vi "Result.Measurement, Screen for Fail or Error.vi"(10 "Meas":T1[](array[typedef]) {"Status" items=["LOG", "PASS", "FAIL", "ERROR"]}, 11 "ResultState In":T3={"State"=enum."Failing", "Code"=0, "Description"=""}) -> (3 "ResultState Out":T3={"State"=enum."Failing", "Code"=0, "Description"=""})   [LabVIEW 2024]
uses:
  <vilib>/KATE/SeqMgr/SeqMgr.Result Info.ctl
  <vilib>/KATE/SeqMgr/SeqMgr.Result State Enum.ctl
  Result.Measurement Item.ctl
  Result.Measurement and Attribute Item Status.ctl
  <vilib>/KATE/SeqMgr/SeqMgr.lvlib
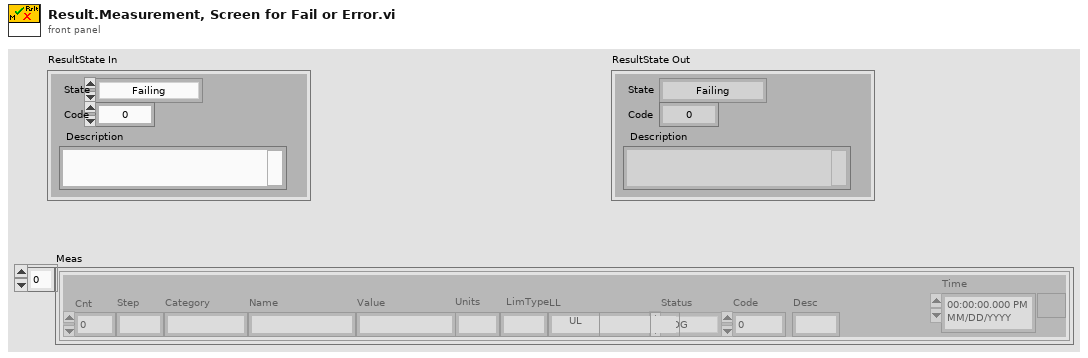
[diagram p1: front panel]
types:
  T1 = typedef "Result.Measurement Item.ctl" = cluster{"Cnt":i32, "Step":string, "Category":string, "Name":string, "Value":string, "Units":string, "LimType":string, "LL":string, "UL":string, "Status":T2, "Code":i32, "Desc":string, "Time":timestamp}
  T2 = typedef "Result.Measurement and Attribute Item Status.ctl" = i32
  T3 = typedef "KATE_Lib.lvlib/SeqMgr.lvlib/SeqMgr.Result Info.ctl" = cluster{"State":T4, "Code":i32, "Description":string}
  T4 = typedef "KATE_Lib.lvlib/SeqMgr.lvlib/SeqMgr.Result State Enum.ctl" = enum16{"None", "Passing", "Failing", "PASS", "FAIL", "ABORT", "ERROR"}
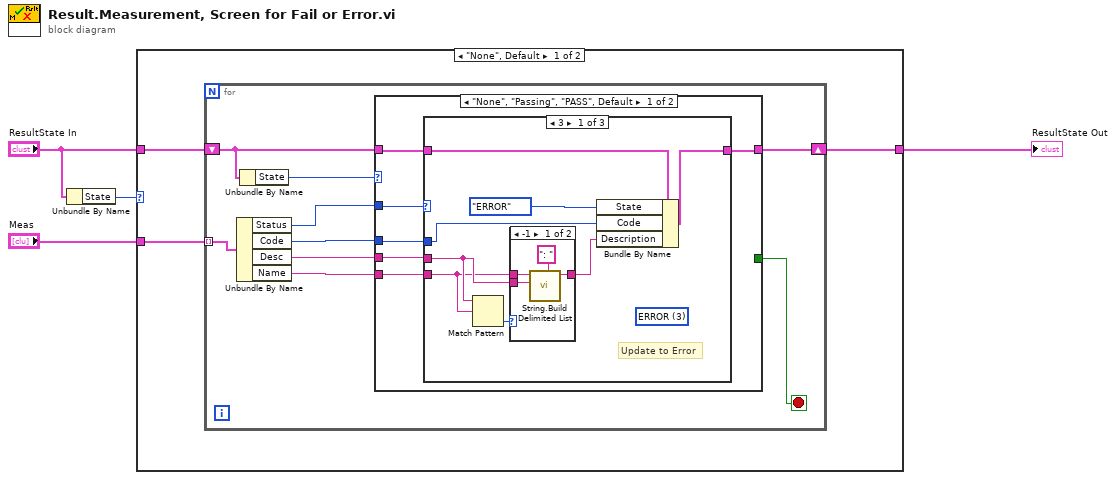
[diagram p0: block diagram]
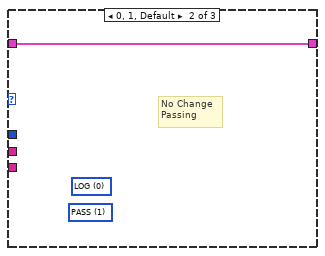
[diagram p3: hidden frame]
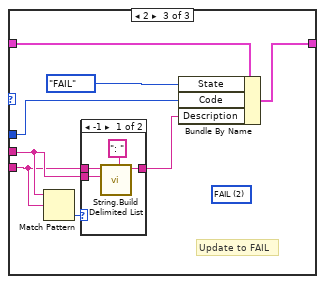
[diagram p4: hidden frame]
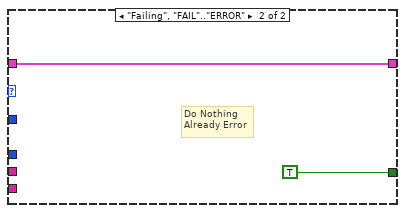
[diagram p6: hidden frame]
diagram:
  n1 = Unbundle By Name("ResultState In") -> ("State"=w3:T4)
  n2 = case shown="\"None\", Default" w3 {
    tunnel: "Meas" -> [w7 _]
    tunnel: "ResultState In" -> [w6 w52]
    tunnel: [w5 w52] -> w1
    frame "None", Default {
      n3 = for {
        tunnel: w7 -> [w16] mode=indexing
        shift-right: [w10] -> w5
        shift-left: w6 -> [w14]
        stop <- w9 stop-if-true
        n4 = Unbundle By Name(w16) -> ("Status"=w13:T2, "Code"=w12:i32, "Desc"=w11:string, "Name"=w8:string)
        n5 = Unbundle By Name(w14) -> ("State"=w15:T4)
        n6 = case shown="\"None\", \"Passing\", \"PASS\", Default" w15 {
          tunnel: w14 -> [w22 w50]
          tunnel: [_ TRUE] -> w9
          tunnel: [w18 w50] -> w10
          tunnel: w13 -> [w21 _]
          tunnel: w12 -> [w20 _]
          tunnel: w11 -> [w19 _]
          tunnel: w8 -> [w17 _]
          frame "None", "Passing", "PASS", Default {
            n7 = case shown="3" w21 {
              tunnel: w22 -> [w30 w36 w43]
              tunnel: [w29 w36 w42] -> w18
              tunnel: w20 -> [w28 _ w41]
              tunnel: w19 -> [w25 _ w39]
              tunnel: w17 -> [w24 _ w38]
              frame 3 {
                (unwired) T2 3 items=["LOG", "PASS", "FAIL", "ERROR"] ("Status")
                # "Update to Error"
                n8 = Match Pattern(string=w25, regular expression=w24) -> (offset past match=w23:i32)  [unwired: 1 in, 3 out]
                n9 = case shown="-1" w23 {
                  tunnel: [w33 w35] -> w26
                  tunnel: w25 -> [w32 w35]
                  tunnel: w24 -> [w31 _]
                  frame -1 {
                    n10 = call "String.Build Delimited List.vi"("Delimiter"=": ", "New Data"=w32, "Existing Str"=w31) -> ("New Str"=w33:string)  [unwired: 8 in]
                  }
                  frame Default {
                  }
                }
                n11 = Bundle By Name(cluster=w30, "State"=SeqMgr.Result_State_Enum."ERROR", "Code"=w28, "Description"=w26) -> (w29:T3)
              }
              frame 0, 1, Default {
                (unwired) T2 1 items=["LOG", "PASS", "FAIL", "ERROR"] ("Status")
                (unwired) T2 0 items=["LOG", "PASS", "FAIL", "ERROR"] ("Status")
                # "No Change\nPassing"
              }
              frame 2 {
                (unwired) T2 2 items=["LOG", "PASS", "FAIL", "ERROR"] ("Status")
                # "Update to FAIL"
                n12 = Match Pattern(string=w39, regular expression=w38) -> (offset past match=w40:i32)  [unwired: 1 in, 3 out]
                n13 = case shown="-1" w40 {
                  tunnel: [w47 w49] -> w37
                  tunnel: w39 -> [w46 w49]
                  tunnel: w38 -> [w45 _]
                  frame -1 {
                    n14 = call "String.Build Delimited List.vi"("Delimiter"=": ", "New Data"=w46, "Existing Str"=w45) -> ("New Str"=w47:string)  [unwired: 8 in]
                  }
                  frame Default {
                  }
                }
                n15 = Bundle By Name(cluster=w43, "State"=SeqMgr.Result_State_Enum."FAIL", "Code"=w41, "Description"=w37) -> (w42:T3)
              }
            }
          }
          frame "Failing", "FAIL".."ERROR" {
            # "Do Nothing\nAlready Error"
          }
        }
      }
    }
    frame "ERROR" {
      # "Already at error - no change"
    }
  }
  "ResultState Out" <- w1
